vi "check sample fifo load.vi"(10 "samples num":u32, 11 "Refnum in":T1) -> (1 "samples remaining":u32, 2 "Boolean":bool, 3 "Refnum out":T1)   [LabVIEW 2020]
uses:
  Host/SubVIs/Streaming Xvcr FPGA Ref.ctl
  <vilib>/Utility/error.llb/Error Cluster From Error Code.vi
  <vilib>/rvi/errors/niLvFpgaAdjustHostInterfaceError.vi
  <vilib>/rvi/interface/nirviMethod/nirviMethod.xnode
  <vilib>/FPGAPlugInAG/Dynamic/niLvFpga_ReadFifo_Dynamic.vi
  <vilib>/rvi/errors/niLvFpgaMergeErrorWithErrorCode.vi
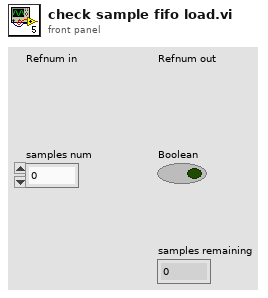
[diagram p1: front panel]
types:
  T1 = typedef "Streaming Xvcr FPGA Ref.ctl" = refnum<k20>
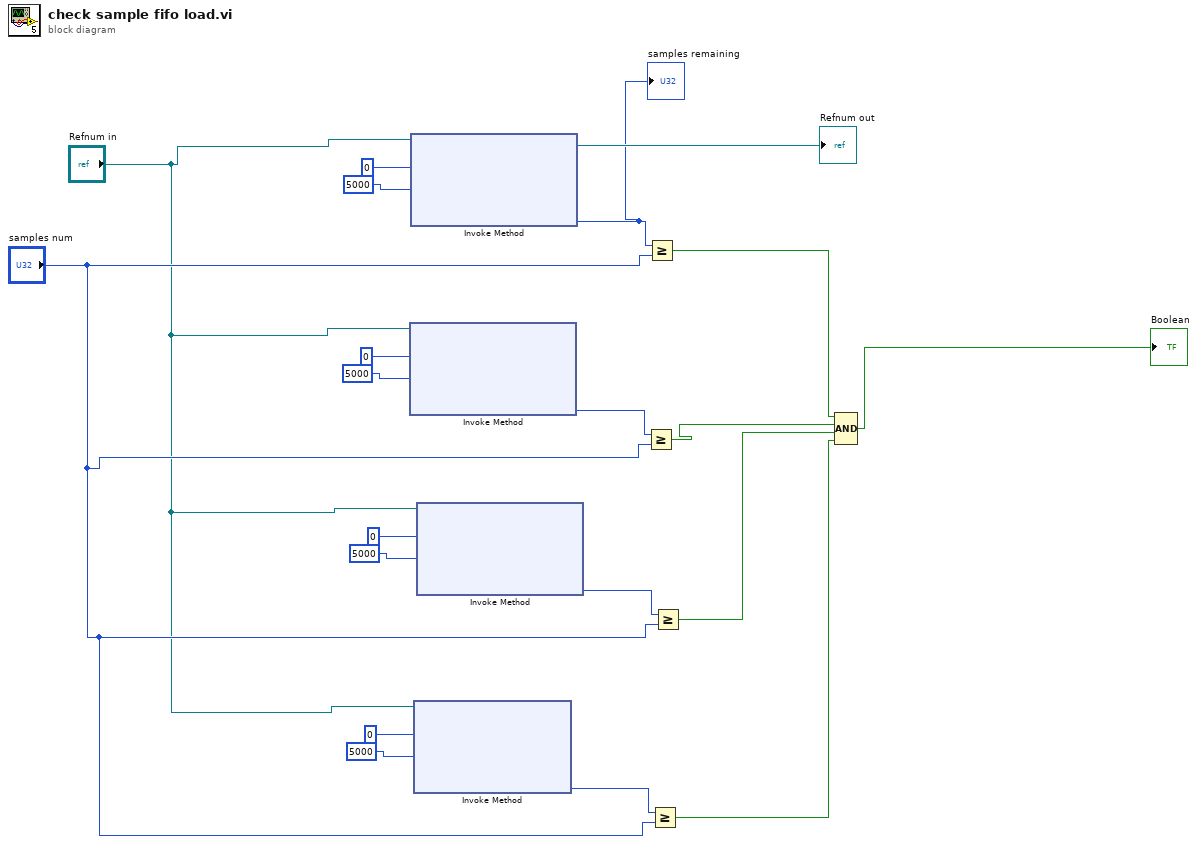
[diagram p0: block diagram]
diagram:
  n1 = xnode "Invoke Method"("FPGA VI Reference In"="Refnum in", "Number of Elements"=u32 0, "Timeout (ms)"=5000) -> ("Elements Remaining"=w15:u32)  [unwired: 1 in, 3 out]
  n2 = xnode "Invoke Method"("FPGA VI Reference In"="Refnum in", "Number of Elements"=u32 0, "Timeout (ms)"=5000) -> ("FPGA VI Reference Out"=→"Refnum out":T1, "Elements Remaining"=w1:u32)  [unwired: 1 in, 2 out]
  "samples remaining" <- w1
  n3 = xnode "Invoke Method"("FPGA VI Reference In"="Refnum in", "Number of Elements"=u32 0, "Timeout (ms)"=5000) -> ("Elements Remaining"=w9:u32)  [unwired: 1 in, 3 out]
  n4 = xnode "Invoke Method"("FPGA VI Reference In"="Refnum in", "Number of Elements"=u32 0, "Timeout (ms)"=5000) -> ("Elements Remaining"=w12:u32)  [unwired: 1 in, 3 out]
  n5 = Greater Or Equal?(x=w15, y="samples num") -> (x >= y?=w6:bool)
  n6 = Greater Or Equal?(x=w1, y="samples num") -> (x >= y?=w7:bool)
  n7 = Greater Or Equal?(x=w9, y="samples num") -> (x >= y?=w4:bool)
  n8 = Greater Or Equal?(x=w12, y="samples num") -> (x >= y?=w5:bool)
  n9 = Compound Arithmetic op=AND(w7, w6, w5, w4) -> (→"Boolean":bool)
